vi "Adjust Text to Fit Rectangle.vi"(0 "VI Name":string, 5 "Number of Rows":i32, 7 "Text settings":T1 {"Alignment" items=["left", "center", "right"]}, 9 "Blank Line 1 text?":bool) -> (4 "Text out":T4)   [LabVIEW 2024, in "Text-Based VI Icon.lvlib"]
uses:
  <vilib>/LabVIEW Icon API/Set Text Icon/Text-Based VI Icon.lvlib
  <vilib>/LabVIEW Icon API/API_Test Settings.ctl
  <vilib>/LabVIEW Icon API/lv_icon/Controls/Alignment.ctl
  <vilib>/LabVIEW Icon API/API_Text Colors.ctl
  <vilib>/LabVIEW Icon API/API_Text.ctl
  <vilib>/LabVIEW Icon API/LabVIEW Icon API.lvlib
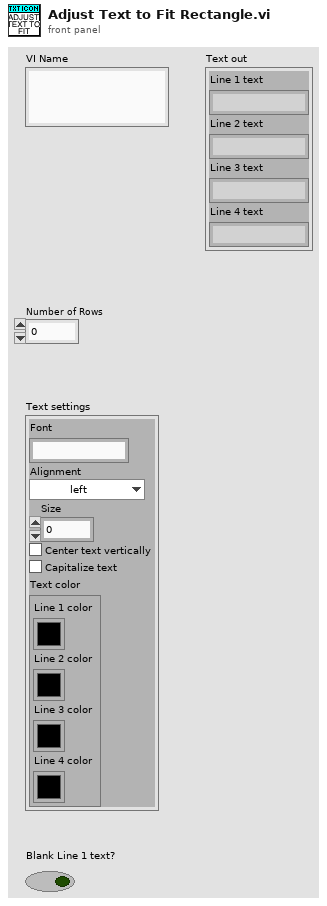
[diagram p1: front panel]
types:
  T1 = typedef "LabVIEW Icon API.lvlib/API_Test Settings.ctl" = cluster{"Font":string, "Alignment":T2, "Size":u8, "Center text":bool, "Capitalize text":bool, "Text color":T3}
  T2 = typedef "Alignment.ctl" = u16
  T3 = typedef "LabVIEW Icon API.lvlib/API_Text Colors.ctl" = cluster{"Line 1 color":u32, "Line 2 color":u32, "Line 3 color":u32, "Line 4 color":u32}
  T4 = typedef "LabVIEW Icon API.lvlib/API_Text.ctl" = cluster{"Line 1 text":string, "Line 2 text":string, "Line 3 text":string, "Line 4 text":string}
  T5 = cluster{"Font Name:":string, "Size":i16, "Strikeout?":bool, "Italic?":bool, "Underline?":bool, "Outline?":bool, "Shadow?":bool, "Bold?":bool}
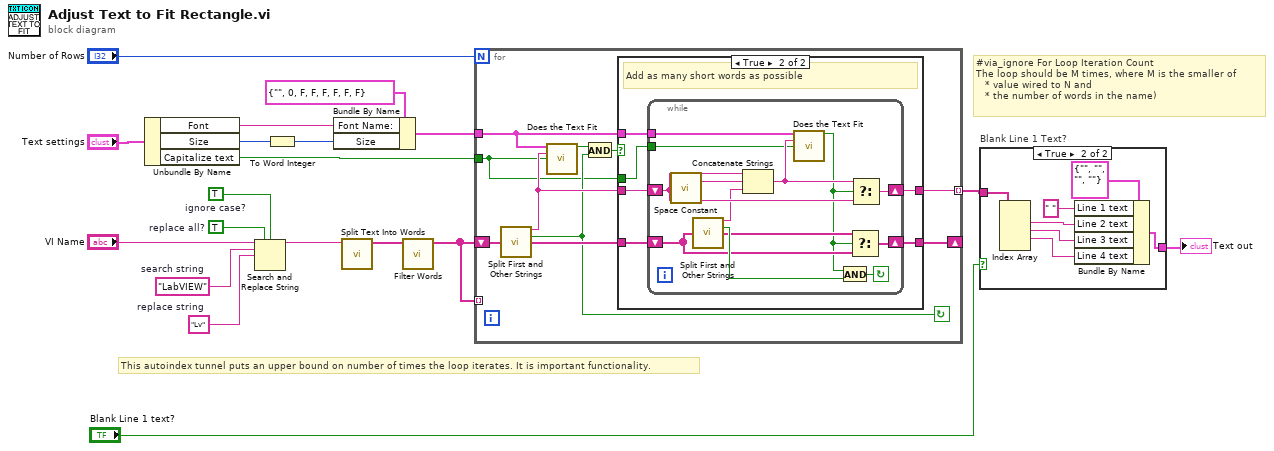
[diagram p0: block diagram]
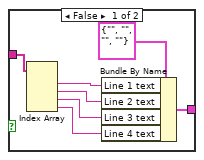
[diagram p2: hidden frame]
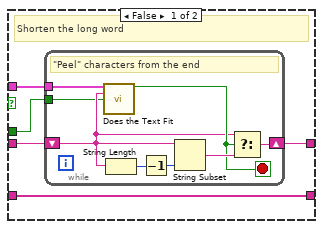
[diagram p3: hidden frame]
diagram:
  w6 = TRUE  # ignore case?
  w7 = TRUE  # replace all?
  w8 = "Lv"  # replace string
  w9 = "LabVIEW"  # search string
  # "This autoindex tunnel puts an upper bound on number of times the loop iterates. It is important functionality."
  # "#via_ignore For Loop Iteration Count\nThe loop should be M times, where M is the smaller of \n   * value wired to N and \n   * the number of words in the name)"
  n1 = Unbundle By Name("Text settings") -> ("Font"=w16:string, "Size"=w15:u8, "Capitalize text"=w12:bool)
  n2 = Search and Replace String(replace all?=w7, case sensitive?=w6, input string="VI Name", search string=w9, replace string=w8) -> (result string=w4:string)  [unwired: 3 in, 3 out]
  n3 = To Word Integer(number=w15) -> (16bit integer=w13:i16)
  n4 = Bundle By Name(cluster=T5 {"Font Name:"="", "Size"=0, "Strikeout?"=FALSE, "Italic?"=FALSE, "Underline?"=FALSE, "Outline?"=FALSE, "Shadow?"=FALSE, "Bold?"=FALSE} ("[user-specified font]"), "Font Name:"=w16, "Size"=w13) -> (w17:T5)
  n5 = call <vilib>:"Split Text Into Words.vi"("VI Name"=w4) -> ("Array"=w11:string[])  [unwired: 10 in]
  n6 = call <vilib>:"Filter Words.vi"("Array in"=w11) -> ("Array out"=w10:string[])  [unwired: 10 in]
  n7 = for {
    N: "Number of Rows" -> [_]
    tunnel: [w21] -> w1 mode=indexing
    tunnel: w17 -> [w28]
    shift-right: [w29] -> _
    shift-left: w10 -> [w25]
    tunnel: w10 -> [_] mode=indexing
    tunnel: w12 -> [w20]
    stop <- w22 continue-if-true
    n8 = call <vilib>:"Split First and Other Strings.vi"("Strings In"=w25) -> ("First String"=w23:string, "One or More Other Strings"=w22:bool, "Other Strings"=w24:string[])  [unwired: 12 in]
    n9 = call <vilib>:"Does the Text Fit.vi"("user-specified font"=w28, "token string"=w23, "Capitalize Text"=w20) -> ("Text Fits"=w27:bool)  [unwired: 12 in]
    n10 = And(x=w27, y=w22) -> (x .and. y?=w26:bool)
    n11 = case shown="True" w26 {
      tunnel: w28 -> [w31 w48]
      tunnel: w23 -> [w33 w47]
      tunnel: [w32 w46] -> w21
      tunnel: [w34 w45] -> w29
      tunnel: w24 -> [w34 w44]
      tunnel: w20 -> [w30 w43]
      frame False {
        # "Shorten the long word"
        n12 = while {
          shift-right: [w40] -> w32
          shift-left: w33 -> [w36]
          tunnel: w31 -> [w42]
          tunnel: w30 -> [w35]
          stop <- w39 stop-if-true
          # "\"Peel\" characters from the end"
          n13 = call <vilib>:"Does the Text Fit.vi"("user-specified font"=w42, "token string"=w36, "Capitalize Text"=w35) -> ("Text Fits"=w39:bool)  [unwired: 12 in]
          n14 = String Length(string=w36) -> (length=w38:i32)
          n15 = Decrement(x=w38) -> (x-1=w37:i32)
          n16 = String Subset(string=w36, length (rest)=w37) -> (substring=w41:string)  [unwired: 1 in]
          n17 = Select(t=w36, s=w39, f=w41) -> (s? t:f=w40:string)
        }
      }
      frame True {
        # "Add as many short words as possible"
        n18 = while {
          shift-right: [w61] -> w46
          shift-left: w47 -> [w58]
          tunnel: w48 -> [w60]
          shift-right: [w56] -> w45
          shift-left: w44 -> [w53]
          tunnel: w43 -> [w49]
          stop <- w55 continue-if-true
          n19 = call <vilib>:"Space Constant.vi"() -> ("String"=w59:string)
          n20 = call <vilib>:"Split First and Other Strings.vi"("Strings In"=w53) -> ("First String"=w51:string, "One or More Other Strings"=w54:bool, "Other Strings"=w52:string[])  [unwired: 12 in]
          n21 = Concatenate Strings(w58, w59, w51) -> (w57:string)
          n22 = call <vilib>:"Does the Text Fit.vi"("user-specified font"=w60, "token string"=w57, "Capitalize Text"=w49) -> ("Text Fits"=w50:bool)  [unwired: 12 in]
          n23 = And(x=w50, y=w54) -> (x .and. y?=w55:bool)
          n24 = Select(t=w52, s=w50, f=w53) -> (s? t:f=w56:string[])
          n25 = Select(t=w57, s=w50, f=w58) -> (s? t:f=w61:string)
        }
      }
    }
  }
  n26 = case "Blank Line 1 Text?" shown="True" "Blank Line 1 text?" {
    tunnel: [w68 w69] -> w3
    tunnel: w1 -> [w63 w71]
    frame False {
      n27 = Index Array(array=w63) -> (element #1=w64:string, element #2=w65:string, element #3=w66:string, element #4=w67:string)  [unwired: 4 in]
      n28 = Bundle By Name(cluster=T4 {"Line 1 text"="", "Line 2 text"="", "Line 3 text"="", "Line 4 text"=""} ("Text out"), "Line 1 text"=w64, "Line 2 text"=w65, "Line 3 text"=w66, "Line 4 text"=w67) -> (w68:T4)
    }
    frame True {
      n29 = Index Array(array=w71) -> (element #1=w73:string, element #2=w74:string, element #3=w75:string)  [unwired: 4 in, 1 out]
      n30 = Bundle By Name(cluster=T4 {"Line 1 text"="", "Line 2 text"="", "Line 3 text"="", "Line 4 text"=""} ("Text out"), "Line 1 text"=" ", "Line 2 text"=w73, "Line 3 text"=w74, "Line 4 text"=w75) -> (w69:T4)
    }
  }
  "Text out" <- w3
